vi "Read Save what.vi"(8 "error in (no error)":errorcluster, 11 "Storage params in":refnum<class "CV-Storage.lvclass">) -> (0 "error out":errorcluster, 2 "Save what?":T1, 3 "Storage params out":refnum<class "CV-Storage.lvclass">)   [LabVIEW 2013, in "CameraVision.lvlib" / "CV-Storage.lvclass"]
uses:
  CV-Storage.lvclass
  CV-Storage.lvclass/CV-Storage.ctl
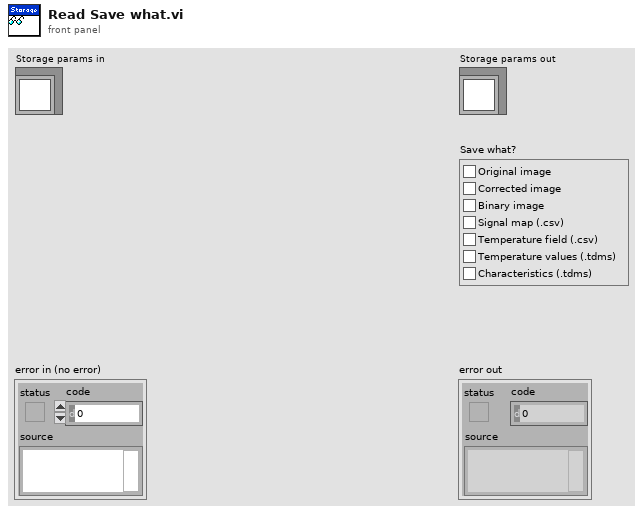
[diagram p1: front panel]
types:
  T1 = cluster{"Original":bool, "Corrected":bool, "Binary":bool, "Temperature":bool, "Characteristics":bool, "Mapping":bool, "TemperatureValues":bool}
  T2 = typedef "CameraVision.lvlib/CV-Storage.lvclass/Storage-types.ctl" = cluster{"Original":bool, "Corrected":bool, "Binary":bool, "Temperature":bool, "Characteristics":bool, "Mapping":bool, "TemperatureValues":bool}
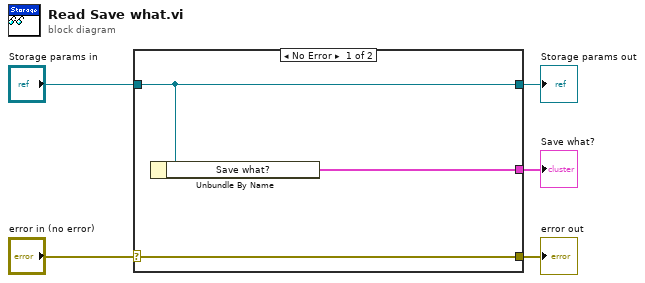
[diagram p0: block diagram]
diagram:
  n1 = case shown="No Error" "error in (no error)" {
    selector: "error in (no error)" -> [w8 w9]
    tunnel: [w8 w9] -> w4
    tunnel: [w7 w10] -> w2
    tunnel: "Storage params in" -> [w7 w10]
    tunnel: [w6 _] -> w1
    frame No Error {
      n2 = Unbundle By Name(w7) -> ("Save what?"=w6:T2)
    }
    frame Error {
    }
  }
  "error out" <- w4
  "Storage params out" <- w2
  "Save what?" <- w1
